vi "ErrorAdd.vi"(1 "source":string="示波器初始化错误") -> (0 "Errorout Souce":string)   [LabVIEW 2018]
panel:
  # "添加错误记录的时间和标记"
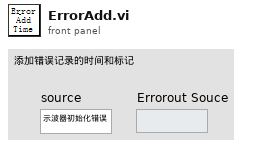
[diagram p1: front panel]
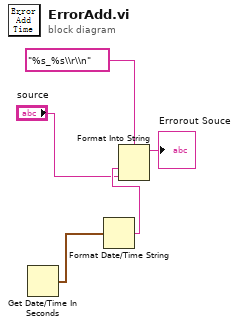
[diagram p0: block diagram]
diagram:
  n1 = Get Date/Time In Seconds() -> (seconds since 1Jan1904=w5:timestamp)
  n2 = Format Date/Time String(seconds (now)=w5) -> (date/time string=w3:string)  [unwired: 2 in]
  n3 = Format Into String(format string="%s_%s\\r\\n" ("格式字符串"), w3, "source") -> (resulting string=→"Errorout Souce":string)  [unwired: 2 in, 1 out]
